vi "write keyword - integer.vi"(8 "error in (no error)":errorcluster, 9 "Value":i32, 10 "keyword":string, 11 "Simulated_Header in":refnum<class "Simulated_Header.lvclass">) -> (0 "error out":errorcluster, 3 "Simulated_Header out":refnum<class "Simulated_Header.lvclass">)   [LabVIEW 2018, in "Simulated_Header.lvclass"]
uses:
  Simulated_Header.lvclass
  Simulated_Header.lvclass/Simulated_Header.ctl
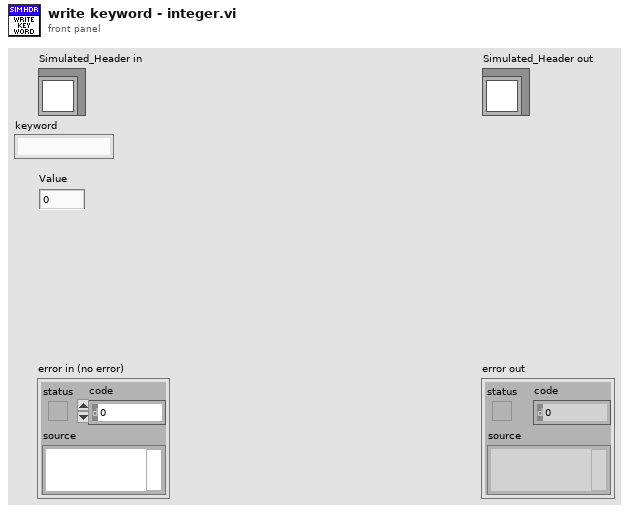
[diagram p1: front panel]
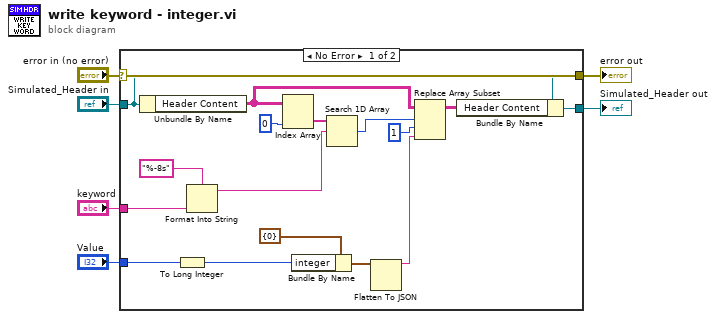
[diagram p0: block diagram]
diagram:
  n1 = case shown="No Error" "error in (no error)" {
    selector: "error in (no error)" -> [w23 w25]
    tunnel: [w23 w25] -> w5
    tunnel: [w16 w24] -> w3
    tunnel: "Simulated_Header in" -> [w17 w24]
    tunnel: "keyword" -> [w8 _]
    tunnel: "Value" -> [w11 _]
    frame No Error {
      n2 = Unbundle By Name(w17) -> ("Header Content"=w20:string[][])
      n3 = To Long Integer(number=w11) -> (32bit integer=w10:i32)
      n4 = Format Into String(format string="%-8s", w8) -> (resulting string=w7:string)  [unwired: 2 in, 1 out]
      n5 = Index Array(array=w20, index (col)=0 ("disabled index (col)")) -> (element=w21:string[])  [unwired: 1 in]
      n6 = Bundle By Name(cluster=cluster{"integer":i32} {"integer"=0}, "integer"=w10) -> (w13:cluster{"integer":i32})
      n7 = Search 1D Array(1D array=w21, element=w7) -> (index of element=w18:i32)  [unwired: 1 in]
      n8 = Flatten To JSON(anything=w13) -> (JSON string=w12:string)  [unwired: 2 in, 1 out]
      n9 = Replace Array Subset(array=w20, new element=w12, index (row)=w18, index (col)=1 ("disabled index (col)")) -> (w15:string[][])
      n10 = Bundle By Name(cluster=w17, "Header Content"=w15) -> (w16:refnum<class "Simulated_Header.lvclass">)
    }
    frame Error {
    }
  }
  "error out" <- w5
  "Simulated_Header out" <- w3
